vi "Write Measurement name.vi"(8 "error in (no error)":errorcluster, 10 "Measurement name":string, 11 "Mag Lab Measurement in":refnum<class "Mag Lab Measurement.lvclass">) -> (0 "error out":errorcluster, 3 "Mag Lab Measurement out":refnum<class "Mag Lab Measurement.lvclass">)   [LabVIEW 2015, in "Mag Lab Measurement.lvclass"]
uses:
  Mag Lab Measurement.lvclass
  Mag Lab Measurement.lvclass/Mag Lab Measurement.ctl
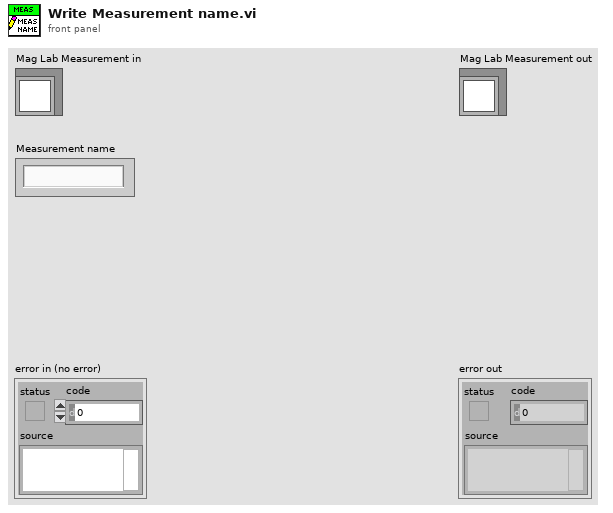
[diagram p1: front panel]
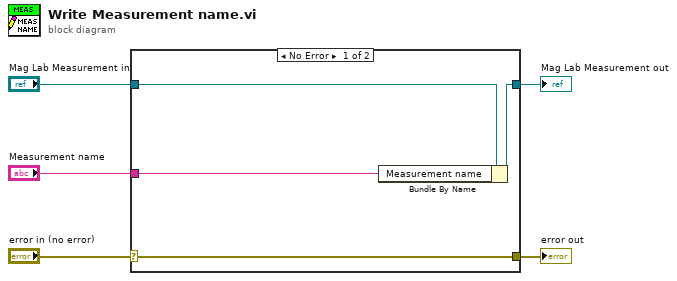
[diagram p0: block diagram]
diagram:
  n1 = case shown="No Error" "error in (no error)" {
    selector: "error in (no error)" -> [w9 w10]
    tunnel: [w9 w10] -> w4
    tunnel: [w7 w11] -> w2
    tunnel: "Mag Lab Measurement in" -> [w8 w11]
    tunnel: "Measurement name" -> [w6 _]
    frame No Error {
      n2 = Bundle By Name(cluster=w8, "Measurement name"=w6) -> (w7:refnum<class "Mag Lab Measurement.lvclass">)
    }
    frame Error {
    }
  }
  "error out" <- w4
  "Mag Lab Measurement out" <- w2
